vi "Emballage_BDD_GVF_Tableau_Historiques.vi"(8 "Error in":errorcluster caption="Error in (no error)", 10 "Tableau historique IN":string[][](array[string])=[["112105740008090004", "01.01.2001 01:01:00", "55", "01234/08-01.01.01", "1", "0"], ["112105740008090006", "01.01.2001 01:01:00", "55", "56789/08-01.01.01", "3", "0"], ["112105740008090007", "01.01.2001 01:01:00", "55", "56789/08-01.01.01", "4", "0"], ["112105740008090007", "01.01.2001 01:01:00", "55", "00123/08-01.01.01", "2", "1"]], 11 "SetGet":T1=enum."get") -> (0 "Error out":errorcluster, 2 "Tableau historique OUT":string[][](array[string])=[["112105740008090004", "01.01.2001 01:01:00", "55", "01234/08-01.01.01", "1", "0"], ["112105740008090006", "01.01.2001 01:01:00", "55", "56789/08-01.01.01", "3", "0"], ["112105740008090007", "01.01.2001 01:01:00", "55", "56789/08-01.01.01", "4", "0"], ["112105740008090007", "01.01.2001 01:01:00", "55", "00123/08-01.01.01", "2", "1"]])   [LabVIEW 2020]
uses:
  Modules/FS/60_FS_Controles/60_FS_SetGet.ctl
panel:
  # "9"
  # "0"
  # "1"
  # "2"
  # "3"
  # "4"
  # "5"
  # "6"
  # "7"
  # "8"
  # "0: NO_VALVE\n1: DATE_EMBALLAGE\n2: VISA_EMBALLAGE\n3: NO_COMMANDE\n4: NO_COMMANDE_LIG\n5: NO_COMMANDE_LIV\n6: NO_COMMANDE_VAL\n7: NO_CARTON\n8: RETOUR_CLIENT\n9: ID_ARTICLE_GPAO"
  # "tableau historique en fonction du type de valve"
  # "0"
  # "1"
  # "2"
  # "3"
  # "4"
  # "5"
  # "6"
  # "7"
  # "8"
  # "9"
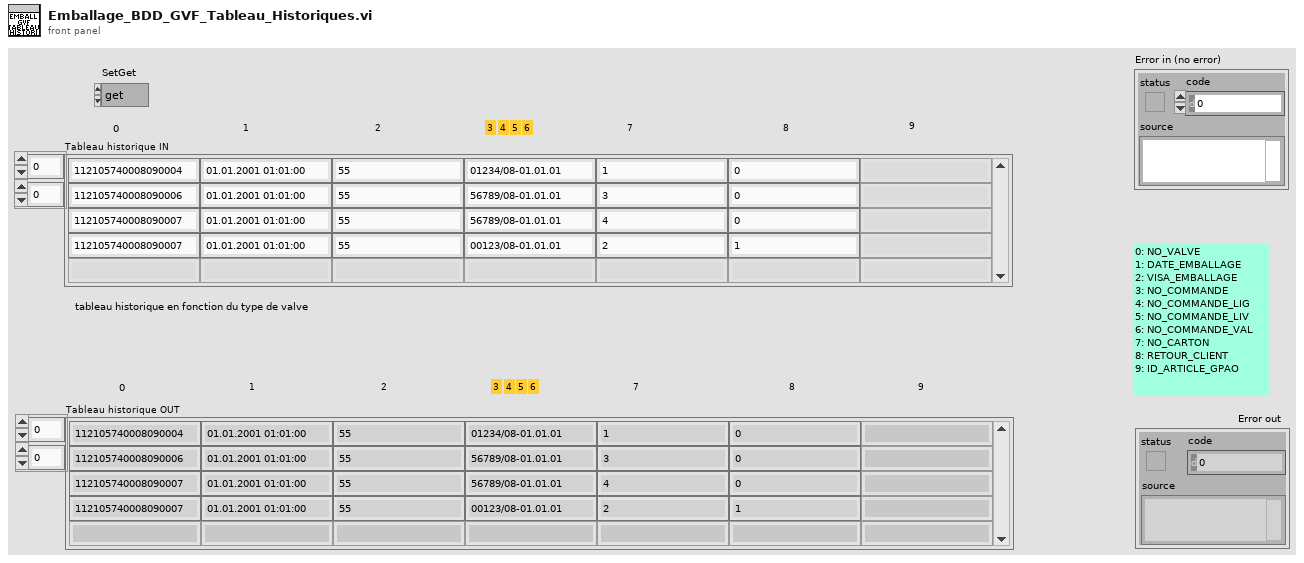
[diagram p1: front panel]
types:
  T1 = typedef "60_FS_SetGet.ctl" = enum16{"set", "get"}
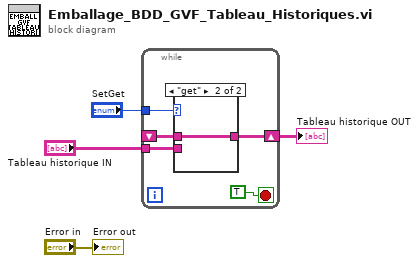
[diagram p0: block diagram]
diagram:
  n1 = while {
    tunnel: "SetGet" -> [w8]
    tunnel: "Tableau historique IN" -> [w6]
    shift-right: [w7] -> w3
    shift-left: _ -> [w5]
    stop <- TRUE stop-if-true
    n2 = case shown="\"get\"" w8 {
      tunnel: [w10 w11] -> w7
      tunnel: w6 -> [w10 _]
      tunnel: w5 -> [_ w11]
      frame "set", Default {
      }
      frame "get" {
      }
    }
  }
  "Tableau historique OUT" <- w3
  "Error out" <- "Error in"
